vi "Write_control_in_stream.vi"(9 "Value":variant, 10 "Required_control_name":string="stop", 11 "reference":refnum<vi>) -> (3 "reference out":refnum<vi>)   [LabVIEW 2012]
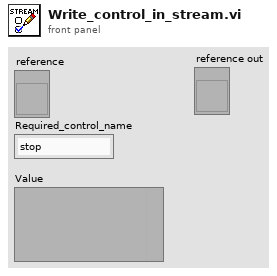
[diagram p1: front panel]
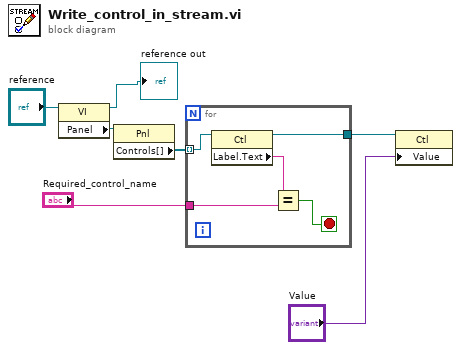
[diagram p0: block diagram]
diagram:
  n1 = property class="VI"(reference="reference") -> (reference out=→"reference out":refnum<vi>, "Panel"=w5:refnum<vi>)  [unwired: 1 in, 1 out]
  n2 = property class="Pnl"(reference=w5) -> ("Controls[]"=w6:refnum<vi>[])  [unwired: 1 in, 2 out]
  n3 = for {
    tunnel: w6 -> [w12] mode=indexing
    tunnel: [w9] -> w7
    tunnel: "Required_control_name" -> [w8]
    stop <- w10 stop-if-true
    n4 = property class="Ctl"(reference=w12) -> (reference out=w9:refnum<vi>, "Label.Text"=w11:string)  [unwired: 1 in, 1 out]
    n5 = Equal?(x=w11, y=w8) -> (x = y?=w10:bool)
  }
  n6 = property class="Ctl"(reference=w7, "Value"="Value") -> ()  [unwired: 1 in, 2 out]
